vi "Vision Processing.vi"(4 "error in (no error)":errorcluster, 7 "Image Size":T1=enum."320x240") -> ()   [LabVIEW 2014]
doc: "This VI runs in parallel to other tasks. It gets images from the camera, processes them for color or shape and use that information to affect robot behavior."
uses:
  <vilib>/Rock Robotics/WPI/Camera/WPI_CameraImageSize.ctl
  <vilib>/Rock Robotics/WPI/Camera/WPI_CameraWhite Balance Values.ctl
  <vilib>/Rock Robotics/WPI/Camera/WPI_CameraExposure Values.ctl
  <vilib>/Rock Robotics/WPI/Camera/WPI_CameraFrameRate.ctl
  Robot Global Data.vi
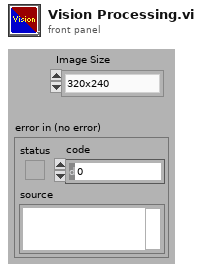
[diagram p1: front panel]
types:
  T1 = typedef "WPI_CameraImageSize.ctl" = enum16{"640x480", "320x240", "160x120", "Custom"}
  T2 = typedef "WPI_CameraFrameRate.ctl" = u32
  T3 = typedef "WPI_CameraExposure Values.ctl" = enum16{"Auto", "Flicker-free 50 Hz", "Flicker-free 60 Hz", "Hold current", "Custom"}
  T4 = typedef "WPI_CameraWhite Balance Values.ctl" = enum16{"Auto", "Fixed indoor", "Fixed outdoor 1", "Fixed outdoor 2", "Fixed fluorescent 1", "Fixed fluorescent 2", "Hold current", "Custom"}
  T5 = typedef "Image Type" = u32
  T6 = typedef "WPI_CameraDevRef.ctl" = cluster{"Camera Address":string, "CameraStatus":errorcluster}
  T7 = typedef "IMAQ Image.ctl" = refnum<image>
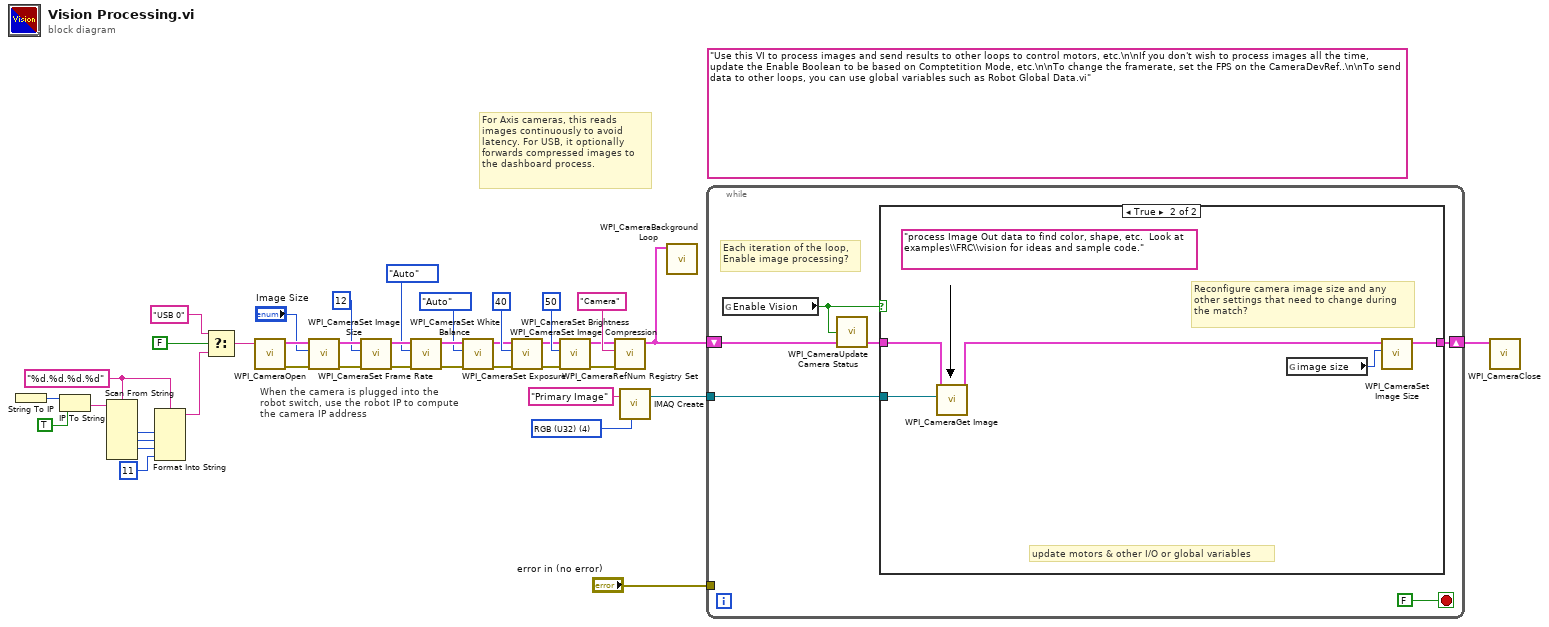
[diagram p0: block diagram]
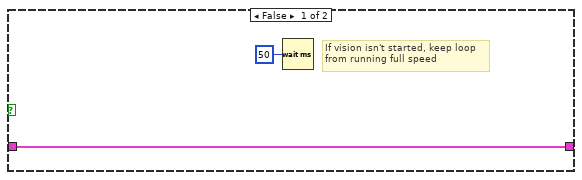
[diagram p2: hidden frame]
diagram:
  w9 = "%d.%d.%d.%d" ("format string")
  (unwired) "Use this VI to process images and send results to other loops to control motors, etc.\n\nIf you don't wish to process images all the time, update the Enable Boolean to be based on Comptetition Mode, etc.\n\nTo change the framerate, set the FPS on the CameraDevRef..\n\nTo send data to other loops, you can use global variables such as Robot Global Data.vi"
  w39 = T5 4 items=["Grayscale (U8)", "Grayscale (I16)", "Grayscale (SGL)", "Complex (CSG)", "RGB (U32)", "HSL (U32)", "RGB (U64)"] ("Image Type")
  # "When the camera is plugged into the\nrobot switch, use the robot IP to compute\nthe camera IP address"
  # "For Axis cameras, this reads\nimages continuously to avoid\nlatency. For USB, it optionally\nforwards compressed images to\nthe dashboard process."
  n1 = String To IP() -> (0:w16:u32)  [unwired: 1 in]
  n2 = IP To String(1:TRUE ("dot notation? (F)"), 2:w16) -> (0:w14:string)
  n3 = Scan From String(format string=w9, input string=w14) -> (output 1=w13:i32, output 2=w12:i32, output 3=w11:i32)  [unwired: 7 in, 3 out]
  n4 = Format Into String(format string=w9, w13, w12, w11, 11 ("Compression")) -> (resulting string=w3:string)  [unwired: 2 in, 1 out]
  n5 = Select(t="USB 0" ("format string"), s=FALSE ("dot notation? (F)"), f=w3) -> (s? t:f=w1:string)
  n6 = call <vilib>:"WPI_CameraOpen.vi"("Camera Address"=w1) -> ("error out"=w27:errorcluster, "CameraDevRef"=w28:T6)  [unwired: 2 in, 7 out]
  n7 = call <vilib>:"WPI_CameraSet Image Size.vi"("error in (no error)"=w27, "Image Size"="Image Size", "CameraDevRef"=w28) -> ("error out"=w26:errorcluster, "CameraDevRef Out"=w29:T6)  [unwired: 1 in, 6 out]
  n8 = call <vilib>:"WPI_CameraSet Frame Rate.vi"("error in (no error)"=w26, "Frame Rate (fps)"=T2 12, "CameraDevRef"=w29) -> ("error out"=w25:errorcluster, "CameraDevRef Out"=w31:T6)  [unwired: 7 out]
  n9 = call <vilib>:"WPI_CameraSet White Balance.vi"("error in (no error)"=w25, "White Balance"=WPI_CameraWhite_Balance_Values."Auto", "CameraDevRef"=w31) -> ("error out"=w24:errorcluster, "CameraDevRef Out"=w30:T6)  [unwired: 1 in, 6 out]
  n10 = call <vilib>:"WPI_CameraSet Exposure.vi"("error in (no error)"=w24, "Exposure"=WPI_CameraExposure_Values."Auto", "CameraDevRef"=w30) -> ("error out"=w23:errorcluster, "CameraDevRef Out"=w33:T6)  [unwired: 1 in, 6 out]
  n11 = call <vilib>:"WPI_CameraSet Image Compression.vi"("error in (no error)"=w23, "Compression"=40, "CameraDevRef"=w33) -> ("error out"=w22:errorcluster, "CameraDevRef Out"=w32:T6)  [unwired: 7 out]
  n12 = call <vilib>:"WPI_CameraSet Brightness.vi"("error in (no error)"=w22, "Brightness"=50, "CameraDevRef"=w32) -> ("error out"=w20:errorcluster, "CameraDevRef Out"=w21:T6)  [unwired: 7 out]
  n13 = call <vilib>:"WPI_CameraRefNum Registry Set.vi"("error in (no error)"=w20, "refnum name"="Camera", "CameraDevRef"=w21) -> ("CameraDevRef"=w8:T6)  [unwired: 8 out]
  n14 = call "IMAQ Create"("Image Name"="Primary Image", "Image Type"=w39) -> ("New Image"=w37:T7)  [unwired: 2 in, 2 out]
  n15 = call <vilib>:"WPI_CameraBackground Loop.vi"("CameraDevRef"=w8) -> ()  [unwired: 11 in]
  n16 = while {
    shift-right: [w44] -> w6
    shift-left: w8 -> [w42]
    tunnel: w37 -> [w43]
    tunnel: "error in (no error)" -> [_]
    stop <- FALSE stop-if-true
    # "Each iteration of the loop,\nEnable image processing?"
    n17 = global read "Robot Global Data.vi" "Enable Vision"() -> (w40:bool)
    n18 = call <vilib>:"WPI_CameraUpdate Camera Status.vi"("CameraDevRef In"=w42, "Enable Vision"=w40) -> ("CameraDevRef Out"=w41:T6)  [unwired: 3 in]
    n19 = case shown="True" w40 {
      tunnel: w43 -> [_ w51]
      tunnel: [w47 w52] -> w44
      tunnel: w41 -> [w47 w49]
      frame False {
        # "If vision isn't started, keep loop\nfrom running full speed"
        n20 = Wait (ms)(milliseconds to wait=u32 50) -> ()  [unwired: 1 out]
      }
      frame True {
        (unwired) "process Image Out data to find color, shape, etc.  Look at examples\\FRC\\vision for ideas and sample code."
        # "update motors & other I/O or global variables"
        # "Reconfigure camera image size and any\nother settings that need to change during\nthe match?"
        n21 = call <vilib>:"WPI_CameraGet Image.vi"("Image"=w51, "CameraDevRef"=w49) -> ("CameraDevRef Out"=w48:T6)  [unwired: 1 in, 8 out]
        n22 = global read "Robot Global Data.vi" "image size"() -> (w50:T1)
        n23 = call <vilib>:"WPI_CameraSet Image Size.vi"("Image Size"=w50, "CameraDevRef"=w48) -> ("CameraDevRef Out"=w52:T6)  [unwired: 2 in, 7 out]
      }
    }
  }
  n24 = call <vilib>:"WPI_CameraClose.vi"("CameraDevRef"=w6) -> ()  [unwired: 1 in, 10 out]
